vi "assignment.vi"() -> ()   [LabVIEW 2022 SP3]
panel:
  out "Numeric 4":dbl
  in  "Numeric 3":dbl
  in  "Numeric 2":dbl
  in  "Numeric":dbl
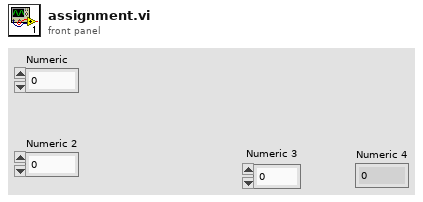
[diagram p1: front panel]
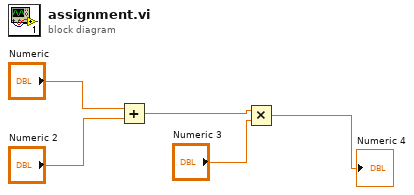
[diagram p0: block diagram]
diagram:
  n1 = Add(x="Numeric", y="Numeric 2") -> (x+y=w3:dbl)
  n2 = Multiply(x=w3, y="Numeric 3") -> (x*y=→"Numeric 4":dbl)
